vi "Tesla Location.vi"() -> ()   [LabVIEW 2020]
uses:
  <vilib>/LVH/i3 JSON/JSON Parsing/Get Object Parameter Files/Get Object Parameter - Array.vi
  <vilib>/LVH/i3 JSON/JSON Parsing/Get Array Value at Index Files/Get Array Value at Index - Object.vi
  <vilib>/LVH/i3 JSON/JSON Parsing/Get Object Parameter Files/Get Object Parameter - String.vi
  <vilib>/LVH/i3 JSON/JSON Parsing/Get Object Parameter Files/Get Object Parameter - Object.vi
  <vilib>/LVH/i3 JSON/JSON Parsing/Get Object Parameter Files/Get Object Parameter - Numeric.vi
  <vilib>/addons/_JKI.lib/REST Client/classes/REST Client/REST Client.lvclass
  <vilib>/LVH/i3 JSON/i3-json.lvlib
panel:
  out "Errors":errorcluster
  in  "Vehicle #":i32
  in  "Tesla Password":string
  in  "Tesla Login Email":string
  out "Timestamp for last update":dbl
  out "longitude":dbl=-97.725479
  out "latitude":dbl=30.409029
  out "Drive state information for vehicle":string="{\"response\":{\"gps_as_of\":1579117675,\"heading\":213,\"latitude\":30.409029,\"longitude\":-97.725479,\"native_latitude\":30.409029,\"native_location_supported\":1,\"native_longitude\":-97.725479,\"native_type\":\"wgs\",\"power\":0,\"shift_state\":null,\"speed\":null,\"timestamp\":1579117676935}}"
  out "JSON array of vehicle data":string="{\"response\":[{\"id\":61186662287574670,\"vehicle_id\":136225104,\"vin\":\"5YJSA1E16FF114124\",\"display_name\":\"Enterprise\",\"option_codes\":\"AD15,MDL3,PBSB,RENA,BT37,ID3W,RF3G,S3PB,DRLH,DV2W,W39B,APF0,COUS,BC3B,CH07,PC30,FC3P,FG31,GLFR,HL31,HM31,IL31,LTPB,MR31,FM3B,RS3H,SA3P,STCP,SC04,SU3C,T3CA,TW00,TM00,UT3P,WR00,AU3P,APH3,AF00,ZCST,MI00,CDM0\",\"color\":null,\"tokens\":[\"3cecbce4c4df802c\",\"f92bf1985118f623\"],\"state\":\"online\",\"in_service\":false,\"id_s\":\"61186662287574670\",\"calendar_enabled\":true,\"api_version\":7,\"backseat_token\":null,\"backseat_token_updated_at\":null},{\"id\":31253816725259093,\"vehicle_id\":1429581797,\"vin\":\"5YJSA1E15GF147326\",\"display_name\":\"Snow White\",\"option_codes\":\"AD15,MDL3,PBSB,RENA,BT37,ID3W,RF3G,S3PB,DRLH,DV2W,W39B,APF0,COUS,BC3B,CH07,PC30,FC3P,FG31,GLFR,HL31,HM31,IL31,LTPB,MR31,FM3B,RS3H,SA3P,STCP,SC04,SU3C,T3CA,TW00,TM00,UT3P,WR00,AU3P,APH3,AF00,ZCST,MI00,CDM0\",\"color\":null,\"tokens\":[\"759624dc39fdb270\",\"b1c01e6323479902\"],\"state\":\"online\",\"in_service\":false,\"id_s\":\"31253816725259093\",\"calendar_enabled\":true,\"api_version\":7,\"backseat_token\":null,\"backseat_token_updated_at\":null}],\"count\":2}"
  # "Leave this at 0 unless you have multiple vehicles"
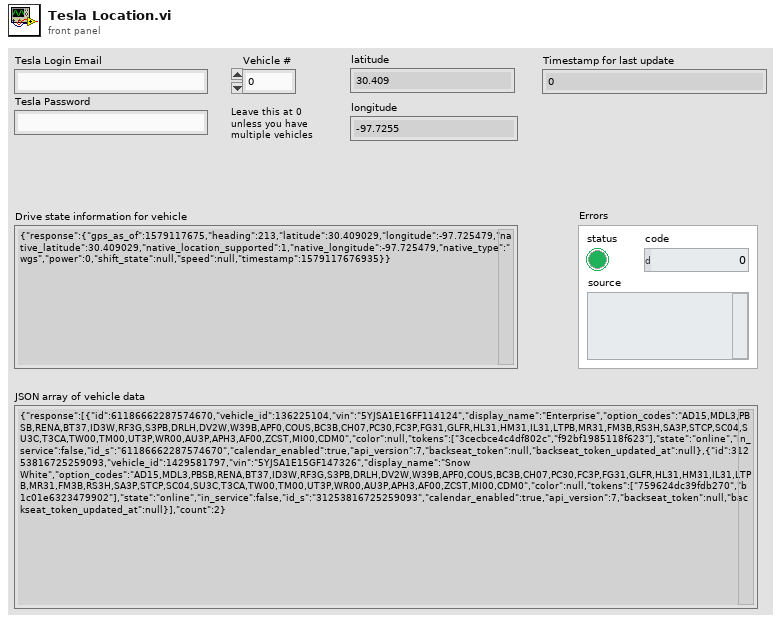
[diagram p1: front panel]
types:
  T1 = typedef "REST Client.lvlib/REST Client.lvclass/HTTP Header.ctl" = cluster{"header":string, "value":string}
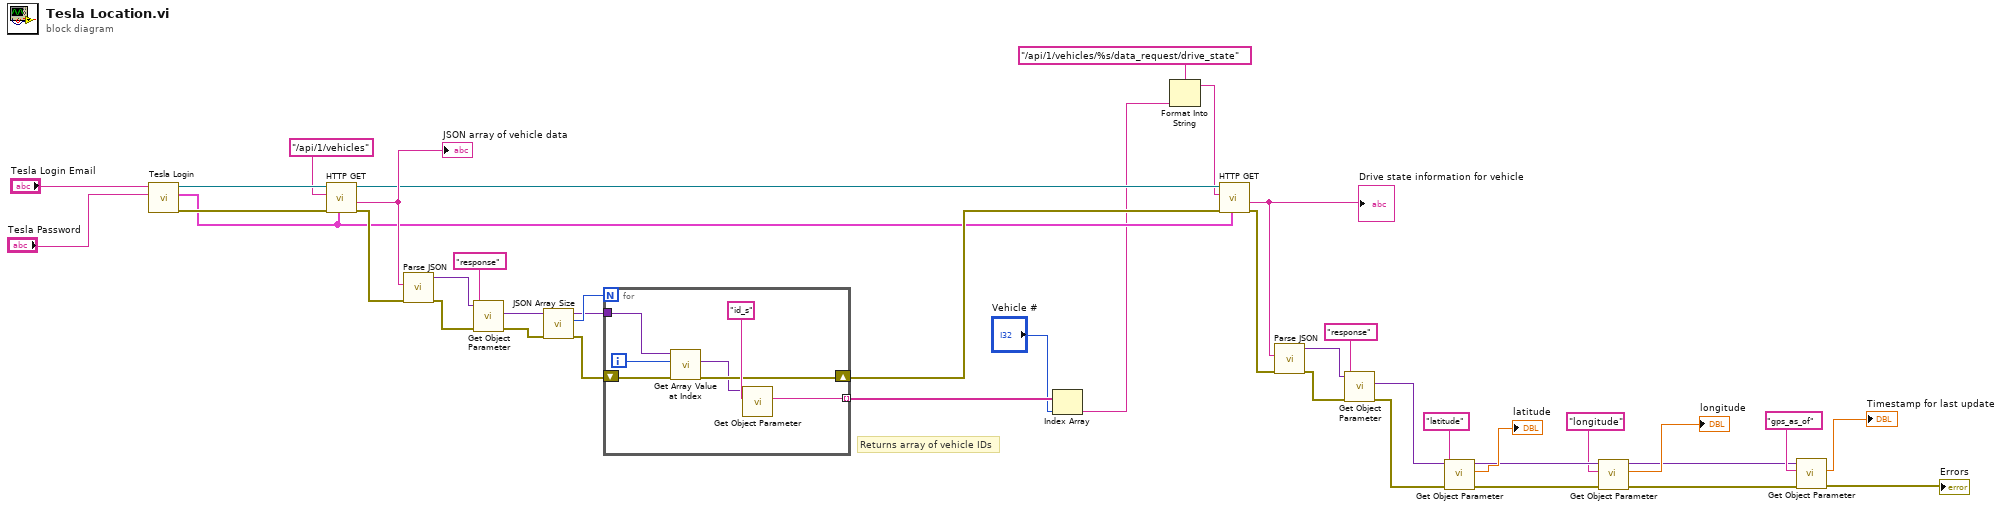
[diagram p0: block diagram]
diagram:
  # "Returns array of vehicle IDs"
  n1 = call "Tesla Login.vi"("password"="Tesla Password", "email"="Tesla Login Email") -> ("error out"=w32:errorcluster, "Tesla Auth Header"=w10:T1[], "REST Client out"=w41:refnum<class "REST Client.lvclass">)  [unwired: 7 in]
  n2 = call-dynamic "HTTP GET.vi"("request specific headers"=w10, "error in (no error)"=w32, "Path"="/api/1/vehicles", "REST Client in"=w41) -> ("error out"=w36:errorcluster, "Response body"=w39:string, "REST Client out"=w29:refnum<class "REST Client.lvclass">)  [unwired: 2 in, 3 out]
  "JSON array of vehicle data" <- w39
  n3 = call <vilib>:"Parse JSON.vi"("error in (no error)"=w36, "JSON String"=w39) -> ("error out"=w35:errorcluster, "JSON Tree"=w26:variant)  [unwired: 6 in, 2 out]
  n4 = call-poly <vilib>:"Get Object Parameter.vi"("error in (no error)"=w35, "Parameter Name"="response", "JSON Tree In (JSON Object)"=w26) -> ("error out"=w34:errorcluster, "JSON Array"=w27:variant)  [unwired: 5 in, 2 out]
  n5 = call <vilib>:"JSON Array Size.vi"("error in (no error)"=w34, "JSON Tree In (JSON Array)"=w27) -> ("error out"=w33:errorcluster, "Array Size"=w37:i32, "JSON Tree Passthrough (JSON Array)"=w25:variant)  [unwired: 7 in]
  n6 = for {
    N: w37 -> [_]
    tunnel: w25 -> [w47]
    shift-right: [w44] -> w28
    shift-left: w33 -> [w45]
    tunnel: [w42] -> w5 mode=indexing
    i -> [w48]
    n7 = call-poly <vilib>:"Get Array Value at Index.vi"("error in (no error)"=w45, "Index"=w48, "JSON Tree In (JSON Array)"=w47) -> ("error out"=w44:errorcluster, "JSON Object"=w43:variant)  [unwired: 5 in, 2 out]
    n8 = call-poly <vilib>:"Get Object Parameter.vi"("Parameter Name"="id_s", "JSON Tree In (JSON Object)"=w43) -> ("String Value"=w42:string)  [unwired: 6 in, 3 out]
  }
  n9 = Index Array(array=w5, index="Vehicle #") -> (element=w4:string)
  n10 = Format Into String(format string="/api/1/vehicles/%s/data_request/drive_state" ("Path 2"), w4) -> (resulting string=w23:string)  [unwired: 2 in, 1 out]
  n11 = call-dynamic "HTTP GET.vi"("request specific headers"=w10, "error in (no error)"=w28, "Path"=w23, "REST Client in"=w29) -> ("error out"=w6:errorcluster, "Response body"=w18:string)  [unwired: 2 in, 4 out]
  "Drive state information for vehicle" <- w18
  n12 = call <vilib>:"Parse JSON.vi"("error in (no error)"=w6, "JSON String"=w18) -> ("error out"=w20:errorcluster, "JSON Tree"=w22:variant)  [unwired: 6 in, 2 out]
  n13 = call-poly <vilib>:"Get Object Parameter.vi"("error in (no error)"=w20, "Parameter Name"="response", "JSON Tree In (JSON Object)"=w22) -> ("error out"=w15:errorcluster, "JSON Object"=w21:variant)  [unwired: 5 in, 2 out]
  n14 = call-poly <vilib>:"Get Object Parameter.vi"("error in (no error)"=w15, "Parameter Name"="latitude", "JSON Tree In (JSON Object)"=w21) -> ("error out"=w12:errorcluster, "Double Value"=→"latitude":dbl, "JSON Tree Out Passthrough"=w14:variant)  [unwired: 5 in, 1 out]
  n15 = call-poly <vilib>:"Get Object Parameter.vi"("error in (no error)"=w12, "Parameter Name"="longitude", "JSON Tree In (JSON Object)"=w14) -> ("error out"=w7:errorcluster, "Double Value"=→"longitude":dbl, "JSON Tree Out Passthrough"=w8:variant)  [unwired: 5 in, 1 out]
  n16 = call-poly <vilib>:"Get Object Parameter.vi"("error in (no error)"=w7, "Parameter Name"="gps_as_of", "JSON Tree In (JSON Object)"=w8) -> ("error out"=→"Errors":errorcluster, "Double Value"=→"Timestamp for last update":dbl)  [unwired: 5 in, 2 out]
